vi "Read Delta Trim Starting Point file.vi"(0 "FIle_Name":string="Delta Trim Values_Starting Point") -> (2 "State":string[](array[string]), 3 "Delta":string[](array[string]))   [LabVIEW 2013]
uses:
  <vilib>/Utility/file.llb/Read From Spreadsheet File (string).vi
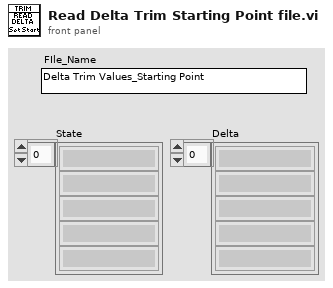
[diagram p1: front panel]
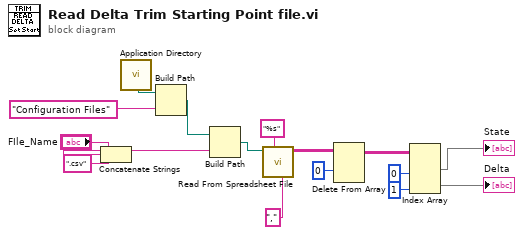
[diagram p0: block diagram]
diagram:
  n1 = Concatenate Strings("FIle_Name", ".csv" ("string")) -> (w7:string)
  n2 = call <vilib>:"Application Directory.vi"() -> ("Application Directory"=w6:path)
  n3 = Build Path(base path=w6, name or relative path="Configuration Files") -> (appended path=w1:path)
  n4 = Build Path(base path=w1, name or relative path=w7) -> (appended path=w4:path)
  n5 = call-poly <vilib>:"Read From Spreadsheet File.vi"("delimiter (\\t)"="," ("delimiter (\\t)"), "format (%s)"="%s", "file path (dialog if empty)"=w4) -> ("all rows"=w14:string[][])  [unwired: 4 in, 4 out]
  n6 = Delete From Array(array=w14, index (row)=0) -> (array with subset deleted=w12:string[][])  [unwired: 2 in, 1 out]
  n7 = Index Array(array=w12, index (col) #1=0 ("disabled index (col)"), index (col) #2=1 ("index (col)")) -> (element #1=→"State":string[], element #2=→"Delta":string[])  [unwired: 2 in]
